vi "LVPortGetTempValue.vi"(0 "pID":string, 1 "Skip Parent Name (t)":bool=TRUE, 2 "Delete Temp (t)":bool=TRUE, 5 "Object ID":i32, 7 "BaseNamepathSrc":string, 9 "Value Type (Or value to update)":variant, 12 "BaseNamepathSrcAr":string[](array[string])) -> (4 "Value":variant, 8 "Object Map Out":T1[](array[typedef]), 15 "Has Invalid Indexing or errored value":bool)   [LabVIEW 2017]
uses:
  Common/ObjectMap/LVPortObjectMapNamepathData.ctl
  Common/ObjectMap/LVPortObjectMapDataTypeEnum.ctl
  Common/ObjectMap/LVPortObjectMapContainerTypeEnum.ctl
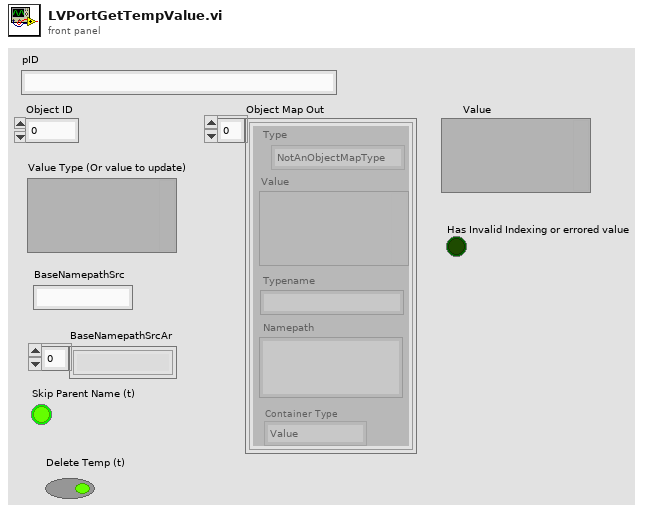
[diagram p1: front panel]
types:
  T1 = typedef "LVPortObjectMapNamepathData.ctl" = cluster{"Type":T2, "Value":variant, "Namepath":string, "Typename":string, "Container Type":T3}
  T2 = typedef "LVPortObjectMapDataTypeEnum.ctl" = enum16{"NotAnObjectMapType", "Real", "Complex", "String", "Boolean"}
  T3 = typedef "LVPortObjectMapContainerTypeEnum.ctl" = enum16{"Value", "Array", "Waveform"}
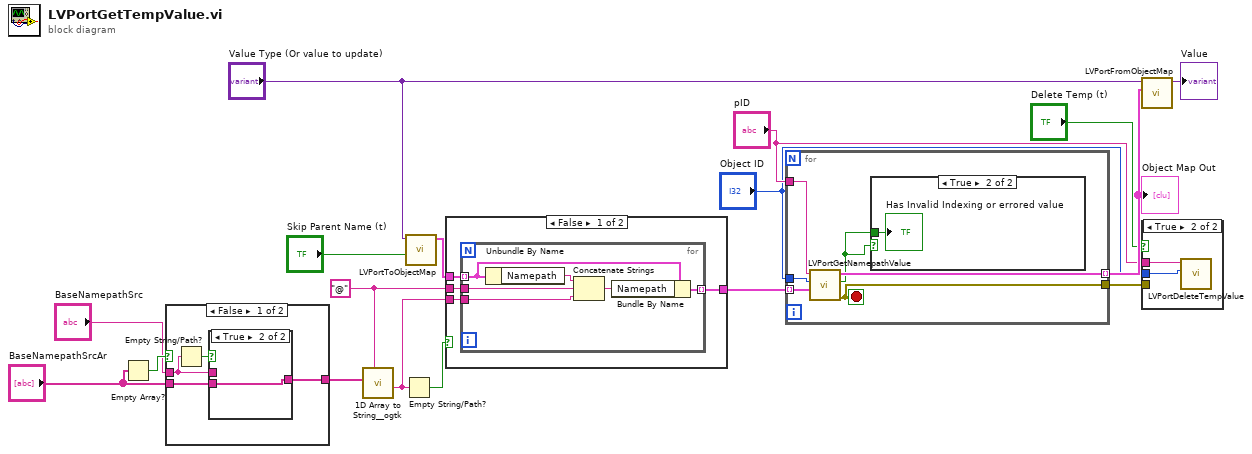
[diagram p0: block diagram]
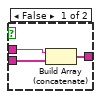
[diagram p5: hidden frame]
diagram:
  w12 = "@" ("delimiter (Tab)")
  n1 = Empty Array?(array="BaseNamepathSrcAr") -> (empty?=w17:bool)
  n2 = case shown="False" w17 {
    tunnel: "BaseNamepathSrc" -> [w21 _]
    tunnel: [w18 w26] -> w14
    tunnel: "BaseNamepathSrcAr" -> [w19 w26]
    frame False {
      n3 = Empty String/Path?(string/path=w21) -> (empty?=w20:bool)
      n4 = case shown="True" w20 {
        tunnel: w21 -> [w24 _]
        tunnel: w19 -> [w23 w25]
        tunnel: [w22 w25] -> w18
        frame False {
          n5 = Build Array (concatenate)(w24, w23) -> (w22:string[])
        }
        frame True {
        }
      }
    }
    frame True {
    }
  }
  n6 = call <userlib>:"1D Array to String__ogtk.vi"("delimiter (Tab)"=w12, "Array of Strings"=w14) -> ("delimited string"=w11:string)  [unwired: 9 in]
  n7 = Empty String/Path?(string/path=w11) -> (empty?=w13:bool)
  n8 = call "LVPortToObjectMap.vi"("Skip Parent Name (t)"="Skip Parent Name (t)", "Value"="Value Type (Or value to update)") -> ("Object map"=w9:T1[])  [unwired: 9 in]
  n9 = case shown="False" w13 {
    tunnel: w9 -> [w30 w37]
    tunnel: w12 -> [w29 _]
    tunnel: w11 -> [w28 _]
    tunnel: [w27 w37] -> w10
    frame False {
      n10 = for {
        tunnel: w30 -> [w36] mode=indexing
        tunnel: w29 -> [w34]
        tunnel: w28 -> [w33]
        tunnel: [w32] -> w27 mode=indexing
        n11 = Unbundle By Name(w36) -> ("Namepath"=w35:string)
        n12 = Concatenate Strings(w35, w34, w33) -> (w31:string)
        n13 = Bundle By Name(cluster=w36, "Namepath"=w31) -> (w32:T1)
      }
    }
    frame True {
    }
  }
  n14 = for {
    tunnel: w10 -> [w43] mode=indexing
    tunnel: "pID" -> [w42]
    tunnel: "Object ID" -> [w41]
    tunnel: [w40] -> w6 mode=indexing
    tunnel: [w39] -> w3
    stop <- w39 stop-if-true
    n15 = call "LVPortGetNamepathValue.vi"("Namepath Data in"=w43, "Object ID"=w41, "pID"=w42) -> ("error out"=w39:errorcluster, "Invalid Indexing or errored value"=w38:bool, "Namepath Data out"=w40:T1)  [unwired: 6 in]
    n16 = case shown="True" w38 {
      tunnel: w38 -> [_ w44]
      frame False {
      }
      frame True {
        "Has Invalid Indexing or errored value" <- w44
      }
    }
  }
  "Object Map Out" <- w6
  n17 = call "LVPortFromObjectMap.vi"("Object Map"=w6, "Type (or value to update)"="Value Type (Or value to update)") -> ("Value"=→"Value":variant)  [unwired: 9 in]
  n18 = case shown="True" "Delete Temp (t)" {
    tunnel: w3 -> [_ _]
    tunnel: "pID" -> [_ w46]
    tunnel: "Object ID" -> [_ w45]
    frame False {
    }
    frame True {
      n19 = call "LVPortDeleteTempValue.vi"("Object ID"=w45, "pID"=w46) -> ()  [unwired: 9 in, 1 out]
    }
  }
